vi "dfd_Extract Output from Sum.vi"(1 "output iwl diff":i16, 2 "x":i64[](array[numeric]) format="%.0x", 4 "output wl":i16, 8 "q_mode":T1=enum."Truncation" caption="round mode") -> (7 "y":i32[](array[numeric]) format="%.0x")   [LabVIEW 2017, in "NI_DigFilter_FXP.lvlib"]
doc: "Actually, the VI convert the integer number from Sum to Output."
uses:
  <vilib>/addons/Digital Filter Design/NI_DigFilter_FXP.lvlib
  <vilib>/addons/Digital Filter Design/_Objects.llb/DFD Round-off Mode.ctl
  <vilib>/addons/Digital Filter Design/NI_DigFilterLicensed.lvlib
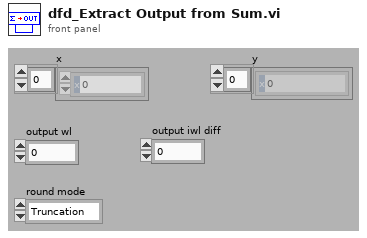
[diagram p1: front panel]
types:
  T1 = typedef "NI_DigFilterLicensed.lvlib/DFD Round-off Mode.ctl" = enum16{"Nearest", "Truncation"}
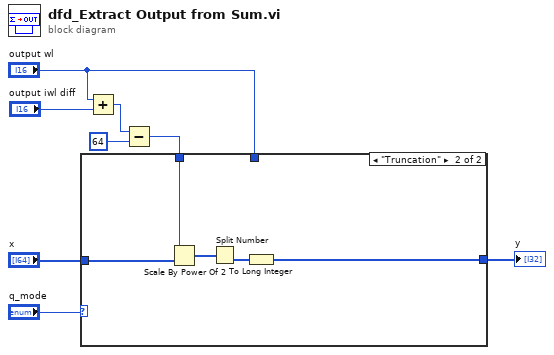
[diagram p0: block diagram]
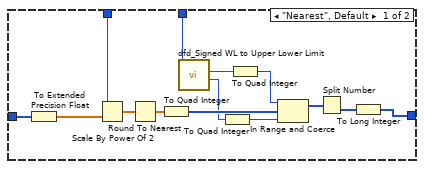
[diagram p2: hidden frame]
diagram:
  n1 = Add(x="output wl", y="output iwl diff") -> (x+y=w1:i16)
  n2 = Subtract(x=w1, y=i16 64) -> (x-y=w7:i16)
  n3 = case shown="\"Truncation\"" "q_mode" {
    tunnel: [w9 w23] -> w4
    tunnel: "x" -> [w22 w27]
    tunnel: w7 -> [w19 w26]
    tunnel: "output wl" -> [w17 _]
    frame "Nearest", Default {
      n4 = To Extended Precision Float(1:w22) -> (0:w21:ext[])
      n5 = Scale By Power Of 2(n=w19, x=w21) -> (x*2^n=w20:ext[])
      n6 = Round To Nearest(number=w20) -> (nearest integer value=w18:ext[])
      n7 = To Quad Integer(1:w18) -> (0:w16:i64[])
      n8 = call <vilib>:"dfd_Signed WL to Upper Lower Limit.vi"("wl"=w17) -> ("lower limit"=w15:i32, "upper limit"=w14:i32)  [unwired: 9 out]
      n9 = To Quad Integer(1:w15) -> (0:w11:i64)
      n10 = To Quad Integer(1:w14) -> (0:w12:i64)
      n11 = In Range and Coerce(upper limit=w12, x=w16, lower limit=w11) -> (coerced(x)=w13:i64[])  [unwired: 1 out]
      n12 = Split Number(x=w13) -> (lo(x)=w10:u32[])  [unwired: 1 out]
      n13 = To Long Integer(number=w10) -> (32bit integer=w9:i32[])
    }
    frame "Truncation" {
      n14 = Scale By Power Of 2(n=w26, x=w27) -> (x*2^n=w24:i64[])
      n15 = Split Number(x=w24) -> (lo(x)=w25:u32[])  [unwired: 1 out]
      n16 = To Long Integer(number=w25) -> (32bit integer=w23:i32[])
    }
  }
  "y" <- w4
